vi "getInheritanceChain.vi"(8 "error in (no error)":errorcluster, 11 "TreeNode in":refnum<class "TreeNode.lvclass">) -> (0 "error out":errorcluster, 2 "Inheritance Chain":string[](array[string]), 3 "TreeNode out":refnum<class "TreeNode.lvclass">)   [LabVIEW 2009, in "TreeNode.lvclass"]
doc: "Returns the inheritance chain."
uses:
  TreeNode.lvclass
  Node/Node.lvclass
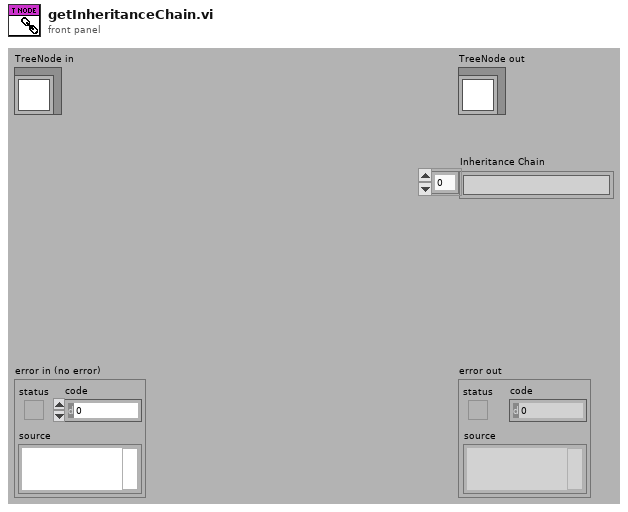
[diagram p1: front panel]
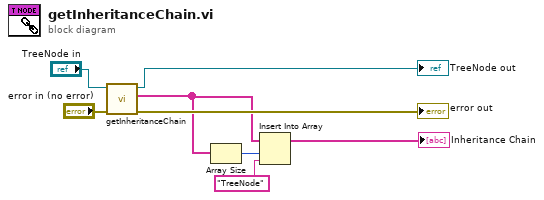
[diagram p0: block diagram]
diagram:
  n1 = call-parent "getInheritanceChain.vi"("error in (no error)"="error in (no error)", "Node in"="TreeNode in") -> ("error out"=→"error out":errorcluster, "Inheritance Chain"=w1:string[], "Node out"=→"TreeNode out":refnum<class "TreeNode.lvclass">)  [unwired: 7 in]
  n2 = Array Size(array=w1) -> (size(s)=w6:i32)
  n3 = Insert Into Array(array=w1, index=w6, new element="TreeNode") -> (→"Inheritance Chain":string[])
